vi "Set Kinematic Parameters.vi"(8 "error in (no error)":errorcluster, 10 "kinematic parameters":T2={"k"=[], "p"=[], "joint type"=enum."Prismatic", "joint coordinate offset"=0.0}, 11 "Link in":refnum<class "Link.lvclass">) -> (0 "error out":errorcluster, 3 "Link out":refnum<class "Link.lvclass">)   [LabVIEW 2013, in "Link.lvclass"]
uses:
  Link.lvclass
  <vilib>/robotics/Kinematics/Link/Joint Type.ctl
  Link.lvclass/Link.ctl
  <vilib>/robotics/Kinematics/Link/NI_Robotics_Link.lvclass
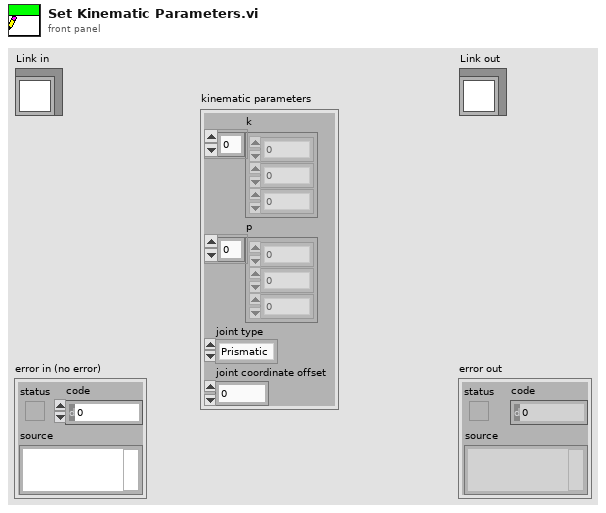
[diagram p1: front panel]
types:
  T1 = typedef "NI_Robotics_Link.lvclass/Joint Type.ctl" = enum16{"Revolute", "Prismatic"}
  T2 = cluster{"k":dbl[], "p":dbl[], "joint type":T1, "joint coordinate offset":dbl}
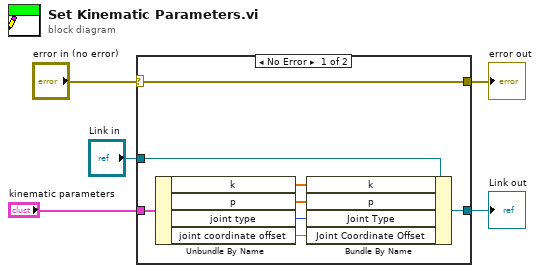
[diagram p0: block diagram]
diagram:
  n1 = case shown="No Error" "error in (no error)" {
    selector: "error in (no error)" -> [w13 w14]
    tunnel: [w13 w14] -> w4
    tunnel: [w11 w15] -> w2
    tunnel: "Link in" -> [w12 w15]
    tunnel: "kinematic parameters" -> [w10 _]
    frame No Error {
      n2 = Unbundle By Name(w10) -> ("k"=w9:dbl[], "p"=w8:dbl[], "joint type"=w7:T1, "joint coordinate offset"=w6:dbl)
      n3 = Bundle By Name(cluster=w12, "k"=w9, "p"=w8, "Joint Type"=w7, "Joint Coordinate Offset"=w6) -> (w11:refnum<class "Link.lvclass">)
    }
    frame Error {
    }
  }
  "error out" <- w4
  "Link out" <- w2
